vi "Get Current State.vi"(8 "error in (no error)":errorcluster, 11 "API In":refnum<class "Interface.lvclass">) -> (0 "error out":errorcluster, 2 "State Messages":refnum<event-registration>, 3 "API out":refnum<class "Interface.lvclass">)   [LabVIEW 2018, in "Scripting.lvlib" / "Actor.lvlib" / "Interface.lvclass"]
uses:
  Interface.lvclass
  State.ctl
  Actor.lvclass
  Interface.lvclass/Interface.ctl
  Get State.ctl
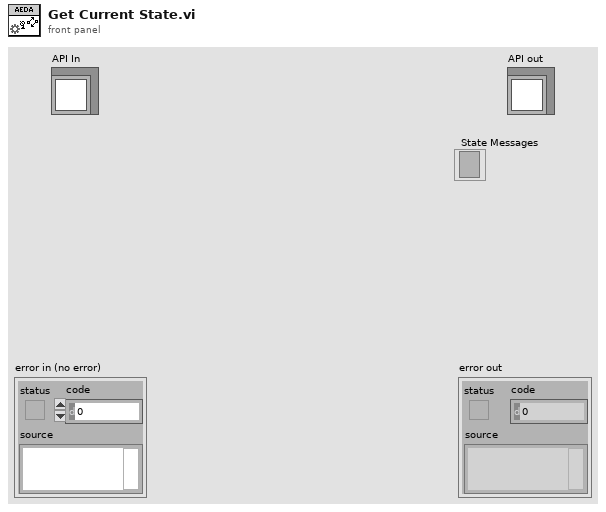
[diagram p1: front panel]
types:
  T1 = typedef "Scripting.lvlib/Actor.lvlib/Actor.lvclass/Get State.ctl" = cluster{"Reply":refnum<user-event>}
  T2 = typedef "Scripting.lvlib/Actor.lvlib/Actor.lvclass/State.ctl" = cluster{"Current State":refnum<class "Actor.lvclass">}
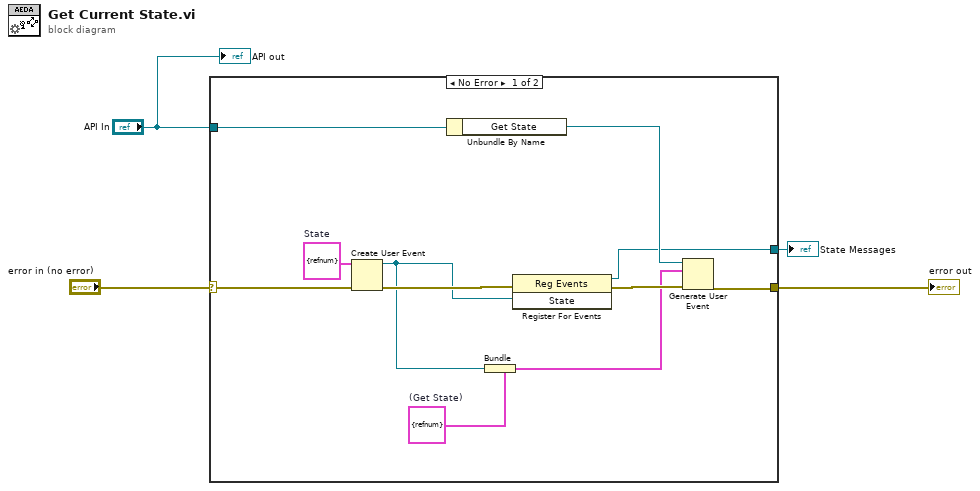
[diagram p0: block diagram]
diagram:
  n1 = case shown="No Error" "error in (no error)" {
    selector: "error in (no error)" -> [w15 w16]
    tunnel: [w14 w16] -> w3
    tunnel: "API In" -> [w13 _]
    tunnel: [w5 _] -> w1
    frame No Error {
      w8 = T1 {"Reply"=refnum}  # (Get State)
      w9 = T2 {"Current State"=refnum}  # State
      n2 = Create User Event(user event datatype=w9, error in=w15) -> (user event=w6:refnum<user-event>, error out=w10:errorcluster)
      n3 = Unbundle By Name(w13) -> ("Get State"=w11:refnum<user-event>)
      n4 = Bundle(cluster=w8, "Reply"=w6) -> (w7:T1)
      n5 = register-events(error in=w10, w6) -> (reference out=w5:refnum<event-registration>, error out=w12:errorcluster)  [unwired: 1 in]
      n6 = Generate User Event(user event=w11, event data cluster=w7, error in=w12) -> (error out=w14:errorcluster)  [unwired: 1 in, 1 out]
    }
    frame Error {
    }
  }
  "error out" <- w3
  "State Messages" <- w1
  "API out" <- "API In"
